vi "Scope_5782_Dual_PID_2channel.vi"() -> ()   [LabVIEW 2013]
uses:
  <vilib>/userdefined/High Color/nirio_resource_hc.ctl
  FPGA/DataMode.ctl
  <vilib>/Analysis/4window.llb/windowTd.ctl
  Host/Scope/controls/power_spectrum_unit.ctl
  Host/Scope5782/Scope/controls/5782_trigger_type.ctl
  Host/Scope/controls/Data_calc_mode.ctl
  Host/Scope/controls/Data_display_mode.ctl
  Host/Scope/controls/Graph_references.ctl
  Host/Scope/controls/graph_controls.ctl
  Host/Scope/controls/Channel_select.ctl
  Host/Communication/response.ctl
  Host/Communication/driver_status.ctl
  Host/Communication/Driver/RemoteConnection/RemoteReferences.ctl
  Host/Communication/Driver/TcpServerDriver/TcpServerDriver.lvclass
  Host/Scope5782/Scope/controls/c_t_type.ctl
  Host/Scope/controls/ScopeMode.ctl
  FPGA/fpga_settings.ctl
  Host/Communication/global_stop.vi
  <vilib>/FPGAPlugInAG/PXIe-7975R/niLvFpga_Open_PXIe-7975R.vi
  <vilib>/rvi/interface/common/dynamic/niFpgaDynamicAddResources.vi
  <vilib>/rvi/interface/common/niFpgaWaitOnOcc.vi
  <vilib>/Utility/error.llb/Error Cluster From Error Code.vi
  <vilib>/rvi/errors/niLvFpgaAdjustHostInterfaceError.vi
  <vilib>/FPGAPlugInAG/Dynamic/niLvFpga_Close_Dynamic.vi
  <vilib>/rvi/interface/nirviOpenFPGA/nirviOpenFPGA.xnode
  FPGA Bitfiles/Dual_PID_2_channel_oCwf2AgGrXE.lvbitx
  <vilib>/rvi/interface/nirviReadWriteControl/nirviReadWriteControl.xnode
  Host/Scope5782/Config/FPGAref_5782.ctl
  <vilib>/rvi/FXPMathLib/FxpInterpret/XNode/nifxpmath_Interpret.xnode
  <vilib>/rvi/interface/nirviMethod/nirviMethod.xnode
  <vilib>/rvi/interface/nirviCloseFPGA/nirviCloseFPGA.xnode
  Host/Utilities/Ticker/Ticker.lvclass
  NiFpgaLv.dll
  <vilib>/rvi/interface/Simulation/niFpgaSimulationCallBeginRW.vi
  Host/Communication/Driver/RemoteConnection/RemoteConnection.lvclass
  <vilib>/FPGAPlugInAG/Dynamic/niLvFpga_WriteFifo_Dynamic.vi
  <vilib>/rvi/errors/niLvFpgaMergeErrorWithErrorCode.vi
  <vilib>/Analysis/NI_AALPro.lvlib
panel:
  in  "Output enabled":bool=TRUE
  in  "unwrap phase":bool
  in  "Kp AM":fxp<+/-,32,4> caption="Kp"
  in  "Kd/T AM":fxp<+/-,32,4> caption="Kd/T"
  in  "Ki*T AM":fxp<+/-,32,4> caption="Ki*T"
  in  "Feedback AM":bool caption="Feedback"
  in  "c(t) AM":bool
  in  "c(t) phase":bool
  in  "Kp":fxp<+/-,32,4>
  in  "Kd/T":fxp<+/-,32,4>
  in  "Ki*T":fxp<+/-,32,4>
  in  "Feedback":bool
  in  "b":fxp<+/-,16,2>
  in  "a":fxp<+/-,16,2>
  in  "Fequency [kHz]":dbl format="%#_8g"
  in  "#bins":i32=1 min=1 max=16
  in  "ch1 DC offset":dbl caption="DC offset\nChannel 1"
  in  "ch0 DC offset":dbl caption="DC offset\nChannel 0"
  in  "Output delay delta":dbl(slide) scale=0.0..6.0
  in  "Output delay":dbl(slide) scale=0.0..6.0
  in  "Chart length":i32=200000
  in  "Trigmode":enum32{"Triggered", "Continuous"}(radio)
  in  "Refence for phase":T1
  in  "Graph_refs":T2
  out "Lower chart":dbl[][](graph)
  out "Upper chart":dbl[][](graph)
  out "Lower graph":i16[][](graph)
  in  "Buffer":T4
  in  "Display":T5
  in  "Output mixer fequency [MHz]":dbl
  in  "Trigger":T6
  in  "Ch1 Q":bool
  in  "Ch1 I":bool
  in  "Ch0 Q":bool
  in  "Ch0 I":bool
  in  "Ch1":bool
  in  "Ch0":bool
  out "stop 2":bool
  in  "Zoom freq X":bool
  in  "Zoom freq Y":bool
  in  "Zoom time Y":bool
  in  "Zoom time X":bool
  in  "Unit":T7
  in  "Window":T8=1 items=["Rectangle"=0, "Hanning"=1, "Hamming"=2, "Blackman-Harris"=3, "Exact Blackman"=4, "Blackman"=5, "Flat Top"=6, "4 Term B-Harris "=7, "7 Term B-Harris"=8, "Low Sidelobe"=9, "Blackman Nuttall"=11, "Triangle"=30, "Bartlett-Hanning"=31, "Bohman"=32, "Parzen"=33, "Welch"=34, "Kaiser"=60, "Dolph-Chebyshev"=61, "Gaussian"=62]
  in  "Samples per 5782 record":i32
  in  "Phase offset (deg)":dbl
  in  "Fequency [MHz]":dbl format="%#_8g"
  in  "Mode":T9
  in  "Mixer freq [MHz]":dbl
  out "freqdata":cluster{"f0":dbl, "df":dbl, "magnitude":dbl[]}[](graph)
  out "Upper graph":i16[][](graph)
  in  "Rumode":bool
  in  "Singleshot":bool
  out "error IO":errorcluster
  in  "stop":bool
  in  "resource name":T10="RIO0"
  out "Clocking Option Configured?":bool
  out "Configured?":bool
  # "FPGA setup"
  # "V"
  # "V"
  # "Output delay"
  # "ns"
  # "Auto Zoom"
  # "Output delay delta"
  # "ps"
  # "Amplitude modulation"
  # "5782"
  # "Phase"
  # "Amplitude"
  # "Simulated data"
  # "FFT"
  # "Auto Zoom"
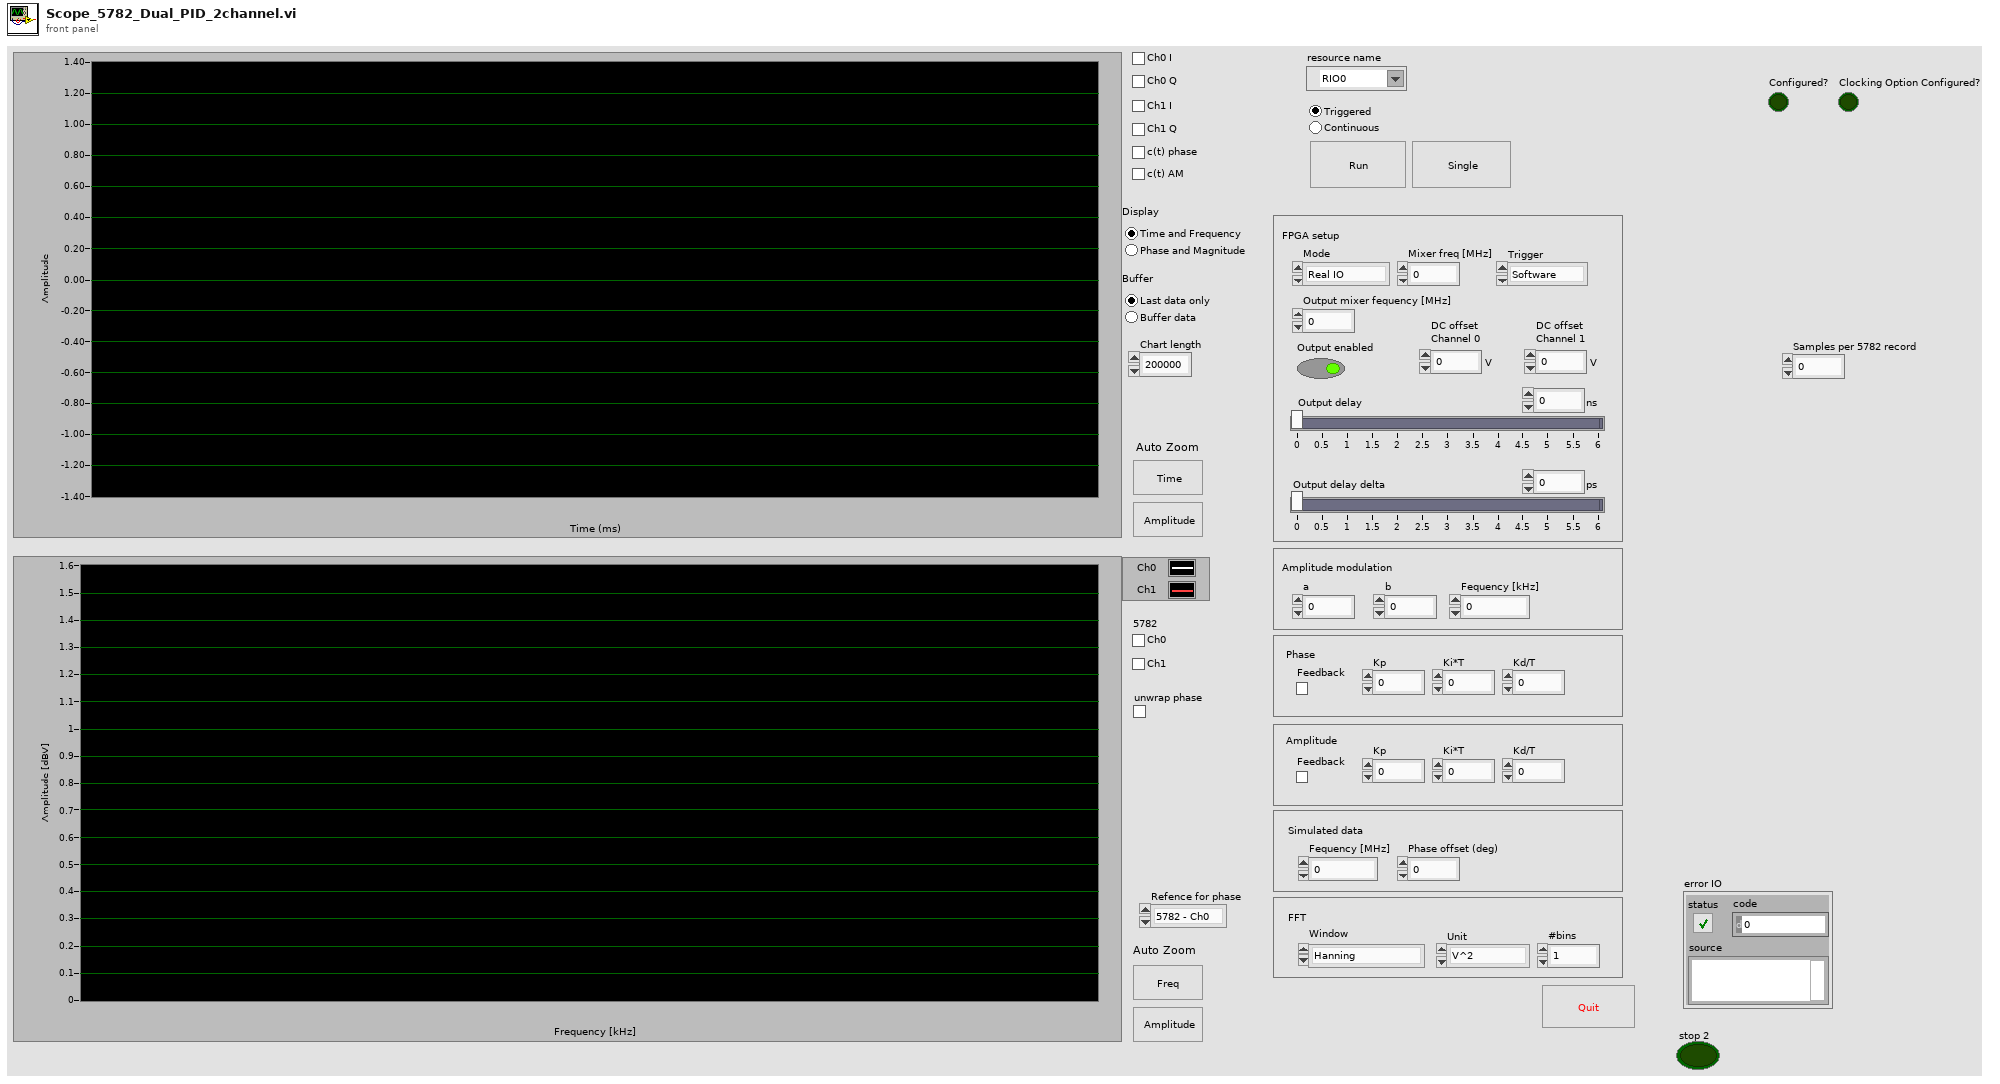
[diagram p1: front panel]
types:
  T1 = typedef "Channel_select.ctl" = enum16{"5782 - Ch0", "5782 - Ch1"}
  T2 = typedef "Graph_references.ctl" = cluster{"upper":T3, "lower":T3, "Freq graph":refnum<vi>}
  T3 = typedef "graph_controls.ctl" = cluster{"Graph":refnum<vi>, "Time btn":refnum<vi>, "Amplitude btn":refnum<vi>, "Chart":refnum<vi>}
  T4 = typedef "Data_display_mode.ctl" = enum32{"Last data only", "Buffer data"}
  T5 = typedef "Data_calc_mode.ctl" = enum32{"Time and Frequency", "Phase and Magnitude"}
  T6 = typedef "5782_trigger_type.ctl" = enum16{"Software", "Trigger input"}
  T7 = typedef "power_spectrum_unit.ctl" = enum16{"V^2", "V", "dBV"}
  T8 = typedef "NI_AALPro.lvlib/windowTd.ctl" = u32
  T9 = typedef "DataMode.ctl" = enum16{"Real IO", "Simulated"}
  T10 = typedef "nirio_resource_hc.ctl" = tag
  T11 = typedef "RemoteConnection.lvclass/RemoteReferences.ctl" = cluster{"a":refnum<vi>, "b":refnum<vi>, "fm":refnum<vi>, "Output delay":refnum<vi>, "Output delay delta":refnum<vi>}
  T12 = typedef "response.ctl" = cluster{"driver status":T13, "Sender":string, "Type":i32, "Variant":variant}
  T13 = typedef "driver_status.ctl" = enum16{"Normal", "Startup", "Connection lost", "Reconnected", "Timeout", "Idle", "Busy"}
  T14 = enum8{"Internal Clock PLL Off", "Internal Clock PLL On (REF IN)", "External Clock (CLK_IN)", "Internal Clock PLL On (IoModSyncClk)"}
  T15 = typedef "message_queue.ctl" = refnum<queue>
  T16 = typedef "FPGAref_5782.ctl" = refnum<k20>
  T17 = typedef "scope_params_5782.ctl" = cluster{"scope mode":T18, "ticker":refnum<class "Ticker.lvclass">, "samples per record":i32, "FPGA ref":T16, "data mode":T9, "5782 Trigger":T6, "Chart length":i32, "RemoteConnection":refnum<class "RemoteConnection.lvclass">, "last phase":dbl[]}
  T18 = typedef "ScopeMode.ctl" = enum16{"Stopped", "Single", "Running", "Continuous"}
  T19 = typedef "c_t_type.ctl" = enum16{"Phase", "AM", "Both", "None"}
  T20 = typedef "fpga_settings.ctl" = enum16{"Feedback Enable", "New FIR coeffs", "FIR shift", "Enable filter", "Set Downsample", "Downsample", "CIC Gain", "Record length", "Trigger samples", "Quiet time", "a_am", "b_am", "Use fixed delay", "fixed sin_fi", "fixed cos_fi", "Ki*Tau", "Kp", "Kd_Tau", "Fi_start", "Fi_delta", "DC_offs 0", "DC_offs 1", "Ki*Tau am", "Kp am", "Kd_Tau am", "Feedback AM"}
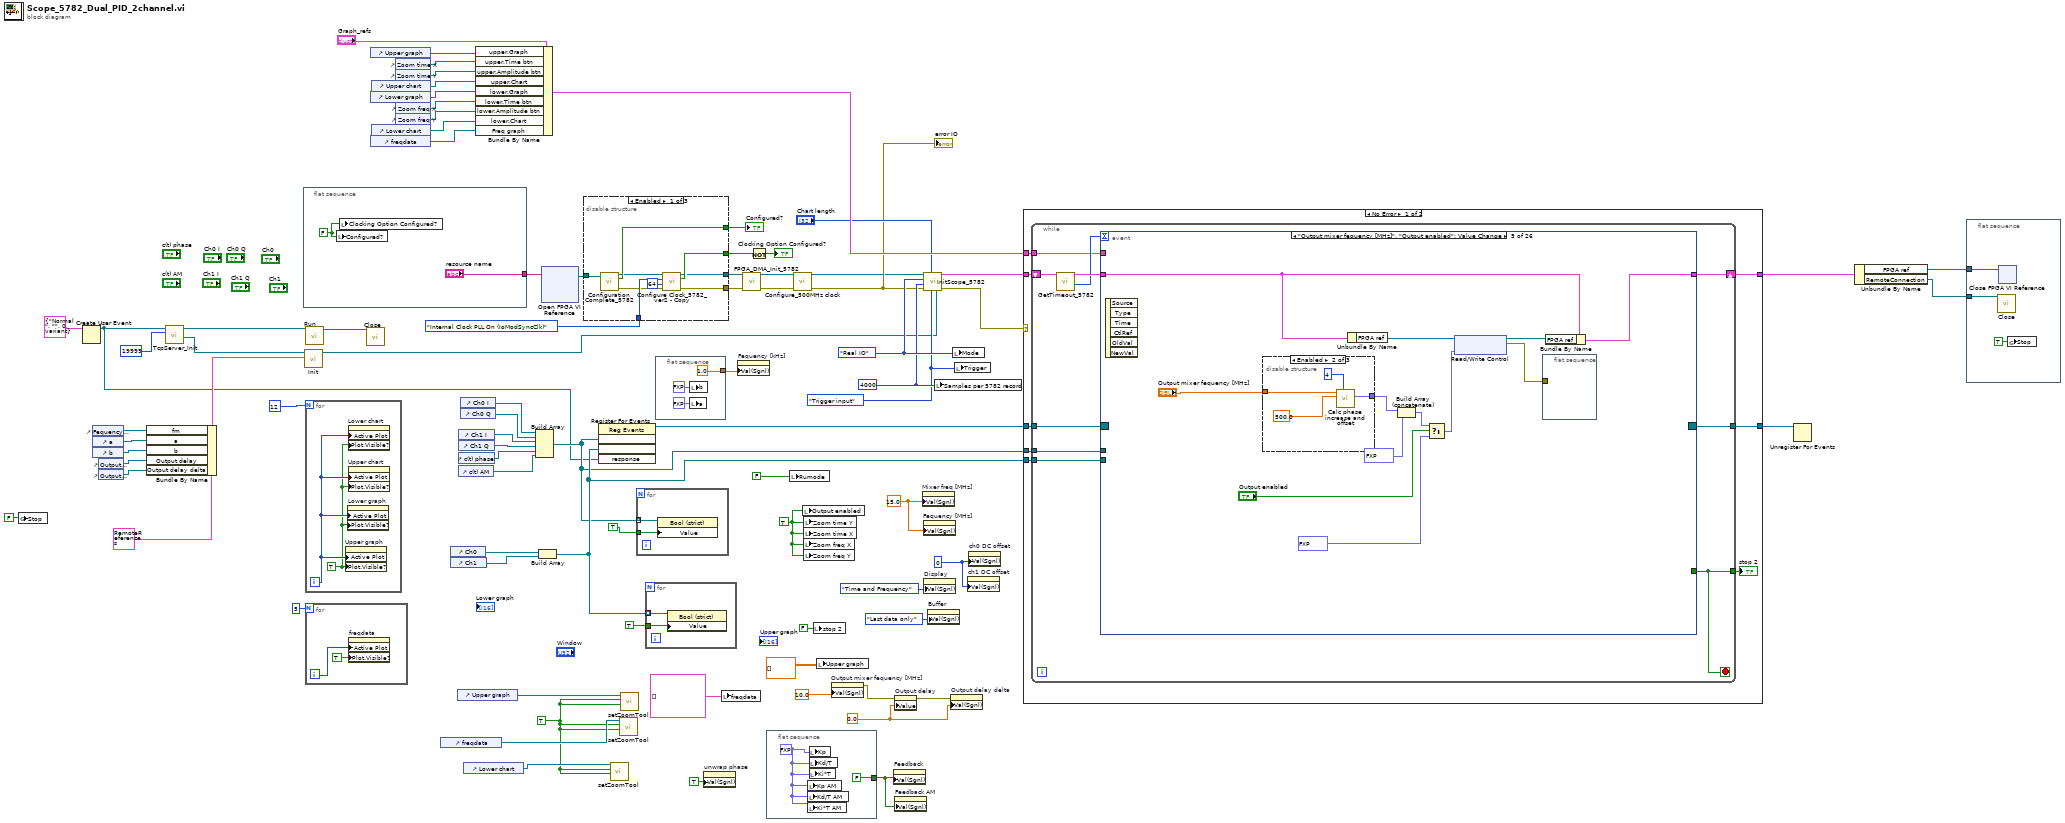
[diagram p0: block diagram]
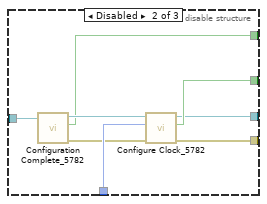
[diagram p2: hidden frame]
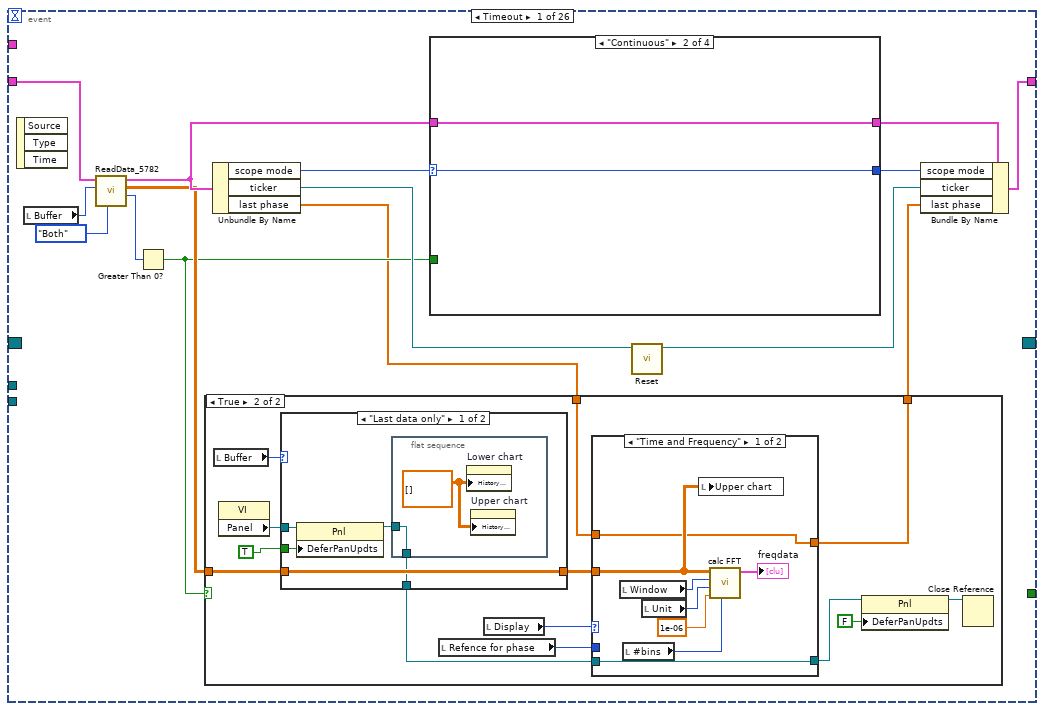
[diagram p4: hidden frame]
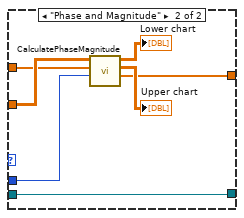
[diagram p7: hidden frame]
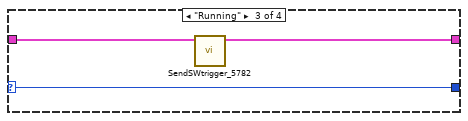
[diagram p9: hidden frame]
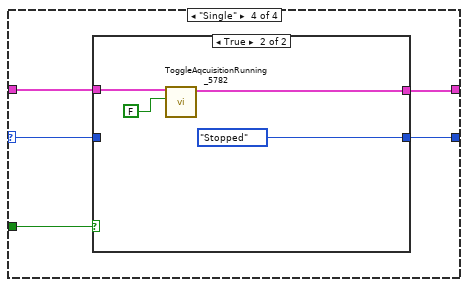
[diagram p10: hidden frame]
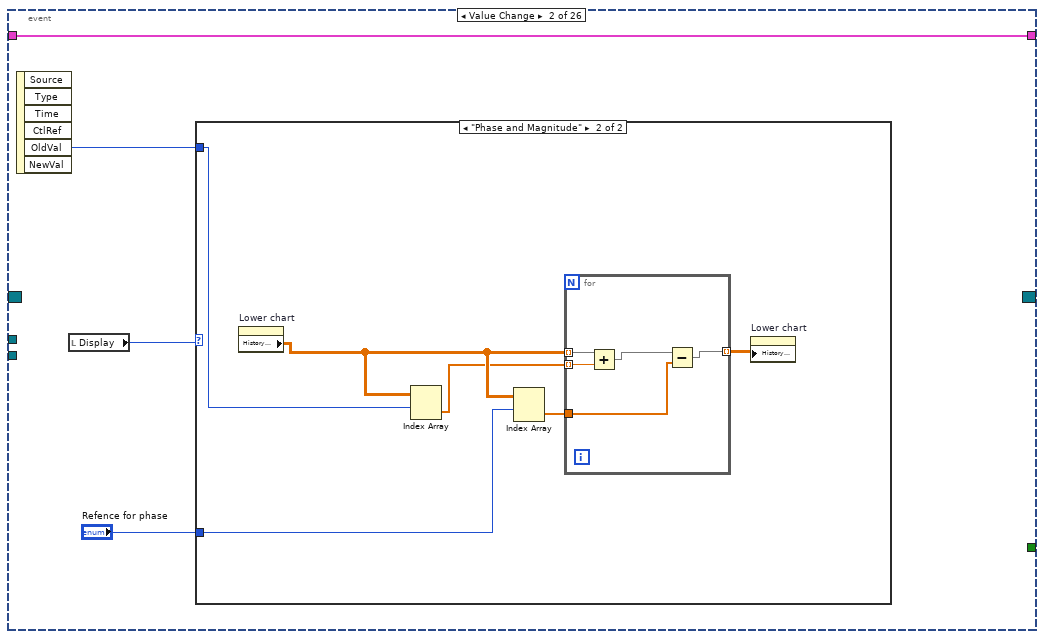
[diagram p12: hidden frame]
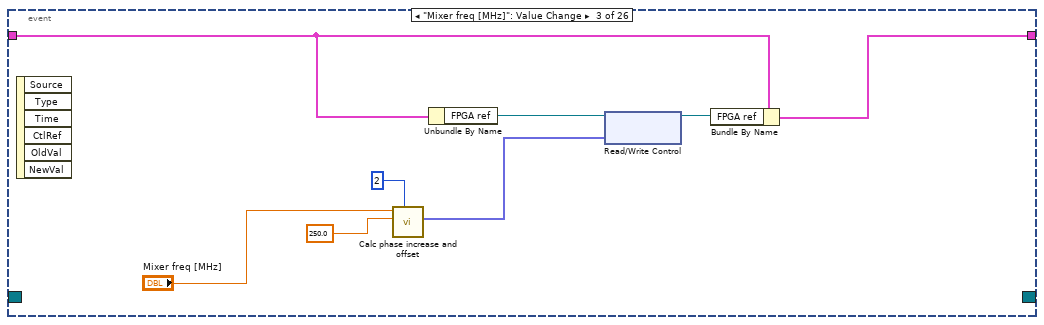
[diagram p14: hidden frame]
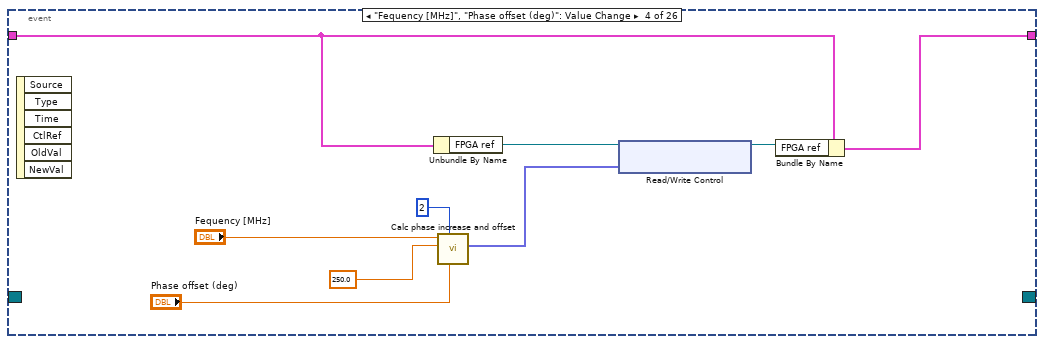
[diagram p15: hidden frame]
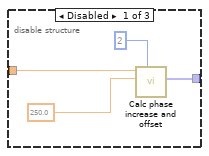
[diagram p16: hidden frame]
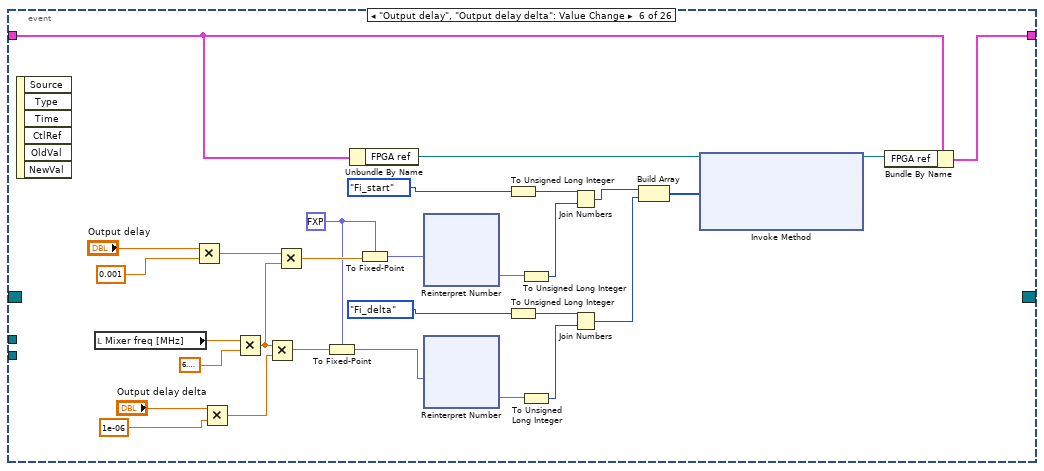
[diagram p18: hidden frame]
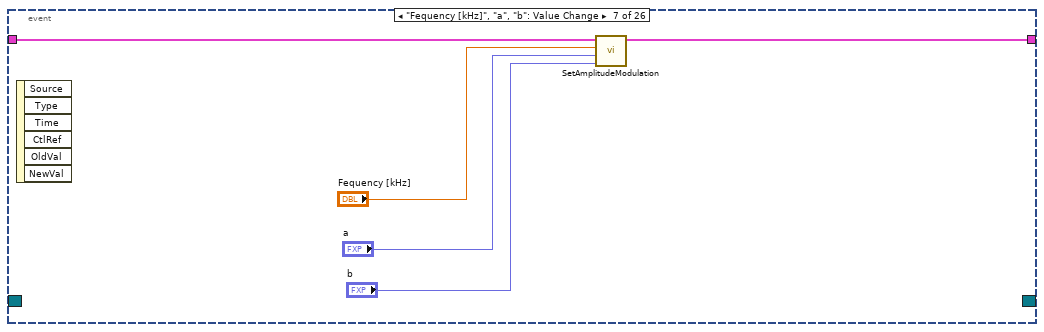
[diagram p19: hidden frame]
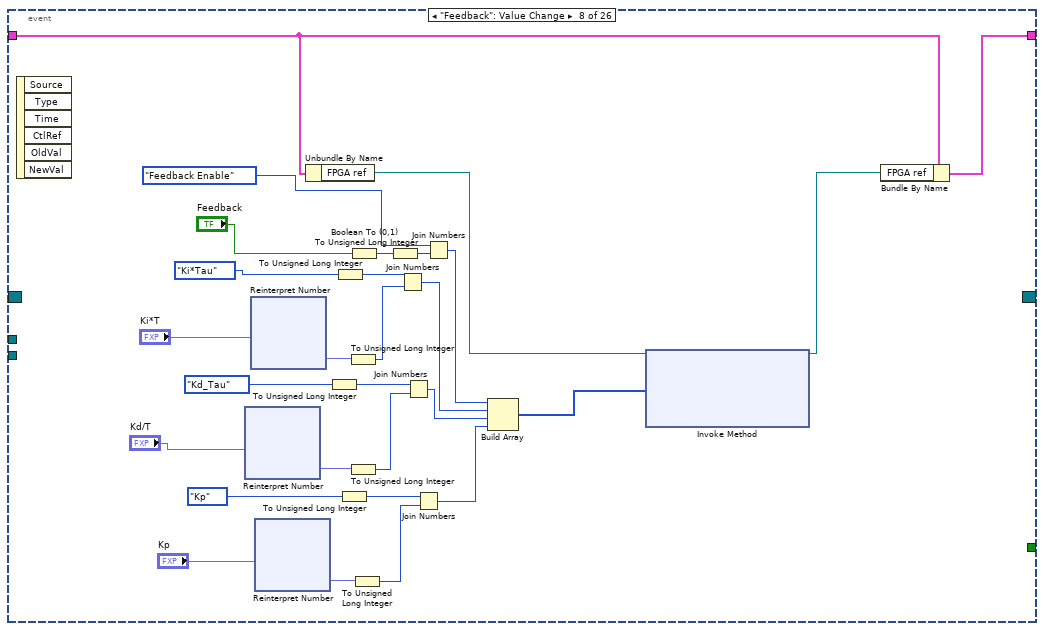
[diagram p20: hidden frame]
diagram:
  w31 = i16 0 ("Value (Signaling)")
  w32 = 0.0 ("Value (Signaling)")
  w55 = 5782_trigger_type."Trigger input" ("Trigger")
  w13 = TRUE ("Zoom  X")
  w1 = TRUE ("Rumode")
  w68 = DataMode."Real IO" ("Mode")
  w57 = 4000 ("Samples to aqcuire")
  w79 = 15.0 ("Mixer requency [MHz]")
  n1 = global write "global_stop.vi" "Stop"(FALSE ("Stop")) -> ()
  n2 = Create User Event(user event datatype=T12 {"driver status"=enum."Normal", "Sender"="", "Type"=0, "Variant"=variant} ("response")) -> (user event=w19:refnum<user-event>)  [unwired: 1 in, 1 out]
  n3 = control-ref of="Fequency [kHz]"() -> (w21:refnum<vi>)
  n4 = control-ref of="a"() -> (w22:refnum<vi>)
  n5 = control-ref of="b"() -> (w20:refnum<vi>)
  n6 = control-ref of="Output delay"() -> (w4:refnum<vi>)
  n7 = control-ref of="Output delay delta"() -> (w3:refnum<vi>)
  n8 = Bundle By Name(cluster=T11 {"a"=refnum, "b"=refnum, "fm"=refnum, "Output delay"=refnum, "Output delay delta"=refnum} ("refs"), "fm"=w21, "a"=w22, "b"=w20, "Output delay"=w4, "Output delay delta"=w3) -> (w29:T11)
  n9 = call "TcpServer_Init.vi"("local port"=u16 19999, "response event"=w19) -> ("Message queue"=w27:T15, "TcpServerDriver"=w24:refnum<class "TcpServerDriver.lvclass">)  [unwired: 8 in]
  n10 = flat-sequence {
    tunnel: ["resource name"] -> w69
    frame #0 {
      w84 = FALSE ("Trigger Acquisition")
      n11 = local write "Configured?"(w84) -> ()
      n12 = local write "Clocking Option Configured?"(w84) -> ()
    }
  }
  n13 = call "Init.vi"("refs"=w29, "server queue"=w27) -> ("RemoteConnection"=w18:refnum<class "RemoteConnection.lvclass">)  [unwired: 9 in]
  n14 = for {
    N: 12 -> [_]
    i -> [w87]
    w86 = TRUE ("Plot.Visible")
    n15 = property on="Upper graph" class="WFGraph (strict)"("Active Plot"=w87, "Plot.Visible?"=w86) -> ()  [unwired: 2 in, 2 out]
    n16 = property on="Lower graph" class="WFGraph (strict)"("Active Plot"=w87, "Plot.Visible?"=w86) -> ()  [unwired: 2 in, 2 out]
    n17 = property on="Lower chart" class="WFChart (strict)"("Active Plot"=w87, "Plot.Visible?"=w86) -> ()  [unwired: 2 in, 2 out]
    n18 = property on="Upper chart" class="WFChart (strict)"("Active Plot"=w87, "Plot.Visible?"=w86) -> ()  [unwired: 2 in, 2 out]
  }
  n19 = for {
    N: 5 -> [_]
    i -> [w88]
    n20 = property on="freqdata" class="WFGraph (strict)"("Active Plot"=w88, "Plot.Visible?"=TRUE ("Plot.Visible")) -> ()  [unwired: 2 in, 2 out]
  }
  n21 = call-dynamic "Run.vi"("BaseDriver in"=w24) -> ("BaseDriver out"=w25:refnum<class "TcpServerDriver.lvclass">)  [unwired: 9 in, 1 out]
  n22 = call-dynamic "Close.vi"("BaseDriver in"=w25) -> ()  [unwired: 9 in, 2 out]
  n23 = control-ref of="Upper graph"() -> (w52:refnum<vi>)
  n24 = control-ref of="Lower graph"() -> (w48:refnum<vi>)
  n25 = control-ref of="freqdata"() -> (w44:refnum<vi>)
  n26 = control-ref of="Upper chart"() -> (w49:refnum<vi>)
  n27 = control-ref of="Lower chart"() -> (w45:refnum<vi>)
  n28 = control-ref of="Zoom time X"() -> (w51:refnum<vi>)
  n29 = control-ref of="Zoom time Y"() -> (w50:refnum<vi>)
  n30 = control-ref of="Zoom freq X"() -> (w47:refnum<vi>)
  n31 = control-ref of="Zoom freq Y"() -> (w46:refnum<vi>)
  n32 = control-ref of="freqdata"() -> (w58:refnum<vi>)
  n33 = control-ref of="Ch0"() -> (w65:refnum<vi>)
  n34 = control-ref of="Ch1"() -> (w66:refnum<vi>)
  n35 = control-ref of="Upper graph"() -> (w59:refnum<vi>)
  n36 = control-ref of="c(t) AM"() -> (w6:refnum<vi>)
  n37 = control-ref of="Ch1 I"() -> (w63:refnum<vi>)
  n38 = control-ref of="Ch1 Q"() -> (w64:refnum<vi>)
  n39 = control-ref of="c(t) phase"() -> (w7:refnum<vi>)
  n40 = control-ref of="Ch0 I"() -> (w61:refnum<vi>)
  n41 = control-ref of="Ch0 Q"() -> (w62:refnum<vi>)
  n42 = control-ref of="Lower chart"() -> (w14:refnum<vi>)
  n43 = Bundle By Name(cluster="Graph_refs", "upper.Graph"=w52, "upper.Time btn"=w51, "upper.Amplitude btn"=w50, "upper.Chart"=w49, "lower.Graph"=w48, "lower.Time btn"=w47, "lower.Amplitude btn"=w46, "lower.Chart"=w45, "Freq graph"=w44) -> (w43:T2)
  n44 = Build Array(w61, w62, w63, w64, w7, w6) -> (w60:refnum<vi>[])
  n45 = Build Array(w65, w66) -> (w71:refnum<vi>[])
  n46 = xnode "Open FPGA VI Reference"("resource name"=w69) -> ("FPGA VI Reference Out"=w37:refnum<k20>)  [unwired: 1 in, 1 out]
  n47 = disable-structure shown="Enabled" {
    disable-tunnel: [w98 w106 _] -> w39
    disable-tunnel: T14."Internal Clock PLL On (IoModSyncClk)" ("Clock Source") -> [w97 w105 _]
    disable-tunnel: [w95 w103 _] -> w38
    disable-tunnel: [w94 w100 w107] -> w12
    disable-tunnel: w37 -> [w92 w102 w107]
    disable-tunnel: [w93 w99 _] -> w35
    frame Enabled {
      n48 = call "Configuration Complete_5782.vi"("FPGA VI Reference in"=w92) -> ("error out"=w96:errorcluster, "Configured?"=w93:bool, "FPGA VI Reference out"=w91:refnum<k20>)  [unwired: 8 in]
      n49 = call "Configure Clock_5782_ver2 - Copy.vi"("error in"=w96, "User Data 1"=u8 64, "Clock Source"=w97, "FPGA VI Reference"=w91) -> ("error out"=w95:errorcluster, "Configuration Error"=w98:bool, "FPGA VI Reference out"=w94:refnum<k20>)  [unwired: 5 in]
    }
    frame Disabled {
      n50 = call "Configuration Complete_5782.vi"("FPGA VI Reference in"=w102) -> ("error out"=w104:errorcluster, "Configured?"=w99:bool, "FPGA VI Reference out"=w101:refnum<k20>)  [unwired: 8 in]
      n51 = call "Configure Clock_5782.vi"("error in"=w104, "Clock Source"=w105, "FPGA VI Reference in"=w101) -> ("error out"=w103:errorcluster, "Configuration Error"=w106:bool, "FPGA VI Reference Out"=w100:T16)  [unwired: 6 in]
    }
    frame Disabled {
    }
  }
  "Configured?" <- w35
  n52 = register-events(w60, w71, w19) -> (reference out=w75:refnum<event-registration>)  [unwired: 2 in, 1 out]
  n53 = call "setZoomTool.vi"("Zoom Y"=w13, "Zoom  X"=w13, "reference"=w14) -> ()  [unwired: 9 in]
  n54 = call "setZoomTool.vi"("Zoom Y"=w13, "Zoom  X"=w13, "reference"=w58) -> ()  [unwired: 9 in]
  n55 = call "setZoomTool.vi"("Zoom Y"=w13, "Zoom  X"=w13, "reference"=w59) -> ()  [unwired: 9 in]
  n56 = for {
    tunnel: w60 -> [w109] mode=indexing
    tunnel: TRUE ("Rumode") -> [w108]
    n57 = property class="Bool (strict)"(reference=w109, "Value"=w108) -> ()  [unwired: 1 in, 2 out]
  }
  n58 = for {
    tunnel: w71 -> [w111] mode=indexing
    tunnel: TRUE ("Rumode") -> [w110]
    n59 = property class="Bool (strict)"(reference=w111, "Value"=w110) -> ()  [unwired: 1 in, 2 out]
  }
  n60 = flat-sequence {
    tunnel: [1.0 ("Value (Signaling)")] -> w30
    frame #0 {
      n61 = local write "b"(fxp<+/-,16,2> 0.0 ("b")) -> ()
      n62 = local write "a"(fxp<+/-,16,2> 1.0 ("a")) -> ()
    }
  }
  n63 = property on="unwrap phase" class="Bool (strict)"("Val(Sgnl)"=TRUE ("Value (Signaling)")) -> ()  [unwired: 2 in, 2 out]
  n64 = local write "freqdata"(cluster{"f0":dbl, "df":dbl, "magnitude":dbl[]}[] [] ("freqdata")) -> ()
  n65 = property on="Fequency [kHz]" class="DigNum (strict)"("Val(Sgnl)"=w30) -> ()  [unwired: 2 in, 2 out]
  n66 = call "FPGA_DMA_Init_5782.vi"("error in (no error)"=w38, "FPGA VI Reference"=w12) -> ("error out"=w10:errorcluster, "FPGA VI Out"=w11:refnum<k20>)  [unwired: 7 in, 1 out]
  n67 = Not(x=w39) -> (.not. x?=→"Clocking Option Configured?":bool)
  n68 = flat-sequence {
    tunnel: [FALSE] -> w5
    frame #0 {
      w115 = fxp<+/-,32,4> 0.0 ("Kp")
      n69 = local write "Kp AM"(w115) -> ()
      n70 = local write "Kd/T AM"(w115) -> ()
      n71 = local write "Ki*T AM"(w115) -> ()
      n72 = local write "Kp"(w115) -> ()
      n73 = local write "Kd/T"(w115) -> ()
      n74 = local write "Ki*T"(w115) -> ()
    }
  }
  n75 = local write "Rumode"(FALSE ("Rumode")) -> ()
  n76 = call "Configure_500MHz clock.vi"("error in"=w10, "FPGA SPI config ref"=w11) -> ("error out"=w9:errorcluster, "FPGA SPI config out"=w8:refnum<k20>)  [unwired: 8 in]
  "error IO" <- w9
  n77 = local write "Output enabled"(w1) -> ()
  n78 = local write "Zoom time Y"(w1) -> ()
  n79 = local write "Zoom time X"(w1) -> ()
  n80 = local write "Zoom freq X"(w1) -> ()
  n81 = local write "Zoom freq Y"(w1) -> ()
  n82 = local write "stop 2"(FALSE ("stop 2")) -> ()
  n83 = local write "Upper graph"(dbl[][] [] ("Timedata")) -> ()
  n84 = property on="Output mixer fequency [MHz]" class="DigNum (strict)"("Val(Sgnl)"=10.0 ("Mixer requency [MHz]")) -> (error out=w33:errorcluster)  [unwired: 2 in, 1 out]
  n85 = property on="Feedback" class="Bool (strict)"("Val(Sgnl)"=w5) -> ()  [unwired: 2 in, 2 out]
  n86 = property on="Output delay" class="Slide (strict)"(error in=w33, "Value"=w32) -> (error out=w34:errorcluster)  [unwired: 1 in, 1 out]
  n87 = property on="Feedback AM" class="Bool (strict)"("Val(Sgnl)"=w5) -> ()  [unwired: 2 in, 2 out]
  n88 = property on="Mixer freq [MHz]" class="DigNum (strict)"("Val(Sgnl)"=w79) -> ()  [unwired: 2 in, 2 out]
  n89 = property on="Fequency [MHz]" class="DigNum (strict)"("Val(Sgnl)"=w79) -> ()  [unwired: 2 in, 2 out]
  n90 = call "InitScope_5782.vi"("RemoteConnection"=w18, "Trigger"=w55, "Chart length"="Chart length", "error in"=w9, "Samples Per Trigger"=w57, "data mode"=w68, "FPGA ref"=w8) -> ("error out"=w15:errorcluster, "scope params"=w83:T17)  [unwired: 3 in]
  n91 = property on="Display" class="RadioBtnsControl (strict)"("Val(Sgnl)"=Data_calc_mode."Time and Frequency" ("Value (Signaling)")) -> ()  [unwired: 2 in, 2 out]
  n92 = property on="Buffer" class="RadioBtnsControl (strict)"("Val(Sgnl)"=enum32{"Last data only", "Buffer data"}."Last data only" ("Value (Signaling)")) -> ()  [unwired: 2 in, 2 out]
  n93 = local write "Samples per 5782 record"(w57) -> ()
  n94 = property on="Output delay delta" class="Slide (strict)"(error in=w34, "Val(Sgnl)"=w32) -> ()  [unwired: 1 in, 2 out]
  n95 = local write "Mode"(w68) -> ()
  n96 = local write "Trigger"(w55) -> ()
  n97 = property on="ch1 DC offset" class="DigNum (strict)"("Val(Sgnl)"=w31) -> ()  [unwired: 2 in, 2 out]
  n98 = property on="ch0 DC offset" class="DigNum (strict)"("Val(Sgnl)"=w31) -> ()  [unwired: 2 in, 2 out]
  n99 = case shown="No Error" w15 {
    tunnel: w83 -> [w124 w498]
    tunnel: [w123 w498] -> w56
    tunnel: w75 -> [w122 w497]
    tunnel: [w121 w497] -> w74
    tunnel: w60 -> [w120 _]
    tunnel: w71 -> [w119 _]
    tunnel: w43 -> [w117 _]
    frame No Error {
      n100 = while {
        shift-right: [w134] -> w123
        shift-left: w124 -> [w133]
        tunnel: w122 -> [w130]
        tunnel: [w129] -> w121
        tunnel: w120 -> [w128]
        tunnel: w119 -> [w127]
        tunnel: [w126] -> w118
        tunnel: w117 -> [w125]
        stop <- w126 stop-if-true
        n101 = call "GetTimeout_5782.vi"("scope in"=w133) -> ("Time left"=w131:i32, "scope out"=w132:T17)  [unwired: 9 in]
        n102 = event shown="[4] \"Output mixer fequency [MHz]\", \"Output enabled\": Value Change" {
          selector: w130 -> [_ _ _ _ _ _ _ _ _ _ _ _ _ _ _ _ _ _ _ _ _ _ _ _ _ _]
          dyn-events: [_ _ _ _ _ _ _ _ _ _ _ _ _ _ _ _ _ _ _ _ _ _ _ _ _ _] -> w129
          timeout: w131 -> [_ _ _ _ _ _ _ _ _ _ _ _ _ _ _ _ _ _ _ _ _ _ _ _ _ _]
          tunnel: [_ _ _ _ _ _ _ _ _ _ _ _ _ _ _ _ _ _ _ _ "stop" _ _ _ _ _] -> w126
          tunnel: w132 -> [w144 w209 w227 w233 w249 w284 w291 w319 w347 w361 w375 w379 w383 w386 w396 w404 w429 w440 w453 w458 w461 w468 w478 w483 w489 w496]
          tunnel: [w147 w209 w225 w232 w248 w283 w290 w318 w346 w360 w374 w378 w382 w385 w393 w401 w429 w440 w453 w457 w461 w468 w478 w483 w489 w496] -> w134
          tunnel: w128 -> [_ _ _ _ _ _ _ _ _ _ _ _ _ _ _ _ w428 _ _ _ _ _ _ _ _ _]
          tunnel: w127 -> [_ _ _ _ _ _ _ _ _ _ _ _ _ _ _ _ _ w430 _ _ _ _ _ _ _ _]
          tunnel: w125 -> [_ _ _ _ _ _ _ _ _ _ _ _ _ _ _ _ _ _ _ _ _ _ _ _ _ w493]
          event Timeout {
            n103 = event-data() -> ()  [unwired: 1 in, 3 out]
            n104 = local read "Buffer"() -> (w138:T4)
            n105 = call "ReadData_5782.vi"("c(t)"=c_t_type."Both", "Buffer mode"=w138, "scope params"=w144) -> ("Num elements"=w140:i32, "data"=w141:dbl[][], "scope params out"=w143:T17)  [unwired: 6 in]
            n106 = Greater Than 0?(x=w140) -> (x > 0?=w139:bool)
            n107 = Unbundle By Name(w143) -> ("scope mode"=w146:T18, "ticker"=w149:refnum<class "Ticker.lvclass">, "last phase"=w137:dbl[])
            n108 = case shown="True" w139 {
              tunnel: w141 -> [_ w160]
              tunnel: w137 -> [w150 w152]
              tunnel: [w150 w151] -> w136
              frame False {
              }
              frame True {
                n109 = local read "Buffer"() -> (w162:T4)
                n110 = property class="VI"() -> ("Panel"=w155:refnum<vi>)  [unwired: 2 in, 2 out]
                n111 = case shown="\"Last data only\"" w162 {
                  tunnel: w160 -> [w168 w172]
                  tunnel: [w168 w172] -> w161
                  tunnel: w155 -> [w167 w171]
                  tunnel: TRUE ("Defer Panel Updates") -> [w165 _]
                  tunnel: [w164 w171] -> w153
                  frame "Last data only" {
                    n112 = property class="Pnl"(reference=w167, "DeferPanUpdts"=w165) -> (reference out=w166:refnum<vi>)  [unwired: 1 in, 1 out]
                    n113 = flat-sequence {
                      tunnel: w166 -> [w169]
                      tunnel: [w169] -> w164
                      frame #0 {
                        w170 = dbl[][] [] ("History Data")
                        n114 = property on="Lower chart" class="WFChart (strict)"("History Data"=w170) -> ()  [unwired: 2 in, 2 out]
                        n115 = property on="Upper chart" class="WFChart (strict)"("History Data"=w170) -> ()  [unwired: 2 in, 2 out]
                      }
                    }
                  }
                  frame "Buffer data" {
                  }
                }
                n116 = local read "Refence for phase"() -> (w159:T1)
                n117 = local read "Display"() -> (w163:T5)
                n118 = case shown="\"Time and Frequency\"" w163 {
                  tunnel: w161 -> [w176 w187]
                  tunnel: w159 -> [_ w184]
                  tunnel: [w175 w183] -> w157
                  tunnel: w153 -> [w175 w183]
                  tunnel: w152 -> [w173 w182]
                  tunnel: [w173 w181] -> w151
                  frame "Time and Frequency" {
                    n119 = local read "Window"() -> (w177:T8)
                    n120 = local read "#bins"() -> (w174:i32)
                    n121 = local read "Unit"() -> (w178:T7)
                    n122 = local write "Upper chart"(w176) -> ()
                    n123 = call "calc FFT.vi"("#bins"=w174, "dt"=1e-06, "Unit"=w178, "Window"=w177, "data"=w176) -> ("Power Spectrum / PSD"=→"freqdata":cluster{"f0":dbl, "df":dbl, "magnitude":dbl[]}[])  [unwired: 6 in]
                  }
                  frame "Phase and Magnitude" {
                    n124 = call "CalculatePhaseMagnitude.vi"("phase reference channel"=w184, "previous phase"=w182, "data"=w187) -> ("last phase"=w181:dbl[], "Magnitude"=→"Upper chart":dbl[][], "Phase"=→"Lower chart":dbl[][])  [unwired: 6 in]
                  }
                }
                n125 = property class="Pnl"(reference=w157, "DeferPanUpdts"=FALSE ("Defer Panel Updates")) -> (reference out=w156:refnum<vi>)  [unwired: 1 in, 1 out]
                n126 = Close Reference(reference=w156) -> ()  [unwired: 1 in, 1 out]
              }
            }
            n127 = case shown="\"Continuous\"" w146 {
              selector: w146 -> [w189 w191 w194 w195]
              tunnel: [w189 w191 w194 w199] -> w145
              tunnel: w143 -> [w188 w190 w193 w197]
              tunnel: [w188 w190 w192 w196] -> w142
              tunnel: w139 -> [_ _ _ w198]
              frame "Stopped" {
              }
              frame "Continuous" {
              }
              frame "Running" {
                n128 = call "SendSWtrigger_5782.vi"("scope in"=w193) -> ("scope out"=w192:T17)  [unwired: 9 in, 1 out]
              }
              frame "Single" {
                n129 = case shown="True" w198 {
                  tunnel: [w200 ScopeMode."Stopped" ("scope mode")] -> w199
                  tunnel: w197 -> [w201 w204]
                  tunnel: [w201 w203] -> w196
                  tunnel: w195 -> [w200 _]
                  frame False {
                  }
                  frame True {
                    n130 = call "ToggleAqcuisitionRunning_5782.vi"("Acquisition running"=FALSE, "scope in"=w204) -> ("scope out"=w203:T17)  [unwired: 8 in, 1 out]
                  }
                }
              }
            }
            n131 = call "Reset.vi"("Ticker in"=w149) -> ("Ticker out"=w148:refnum<class "Ticker.lvclass">)  [unwired: 9 in, 1 out]
            n132 = Bundle By Name(cluster=w142, "scope mode"=w145, "ticker"=w148, "last phase"=w136) -> (w147:T17)
          }
          event Value Change {
            n133 = event-data() -> ("OldVal"=w206:T1)  [unwired: 1 in, 5 out]
            n134 = local read "Display"() -> (w207:T5)
            n135 = case shown="\"Phase and Magnitude\"" w207 {
              tunnel: "Refence for phase" -> [_ w214]
              tunnel: w206 -> [_ w212]
              frame "Time and Frequency", Default {
              }
              frame "Phase and Magnitude" {
                n136 = property on="Lower chart" class="WFChart (strict)"() -> ("History Data"=w213:dbl[][])  [unwired: 2 in, 2 out]
                n137 = Index Array(array=w213, index (row)=w212) -> (element=w211:dbl[])  [unwired: 1 in]
                n138 = Index Array(array=w213, index (row)=w214) -> (element=w215:dbl[])  [unwired: 1 in]
                n139 = for {
                  tunnel: w213 -> [w218] mode=indexing
                  tunnel: w215 -> [w220]
                  tunnel: [w219] -> w210 mode=indexing
                  tunnel: w211 -> [w217] mode=indexing
                  n140 = Add(x=w218, y=w217) -> (x+y=w216:dbl[])
                  n141 = Subtract(x=w216, y=w220) -> (x-y=w219:dbl[])
                }
                n142 = property on="Lower chart" class="WFChart (strict)"("History Data"=w210) -> ()  [unwired: 2 in, 2 out]
              }
            }
          }
          event "Mixer freq [MHz]": Value Change {
            n143 = event-data() -> ()  [unwired: 1 in, 6 out]
            n144 = call "Calc phase increase and offset.vi"("# of DDS"=2, "fclk (MHz)"=250.0 ("fclk (800MHz)"), "f_generated (MHz)"="Mixer freq [MHz]") -> ("Phase out"=w221:fxp<+,64,64>[])  [unwired: 6 in, 2 out]
            n145 = Unbundle By Name(w227) -> ("FPGA ref"=w228:T16)
            n146 = xnode "Read/Write Control"("FPGA VI Reference In"=w228, "Phase 5782"=w221) -> ("FPGA VI Reference Out"=w226:T16)  [unwired: 1 in, 1 out]
            n147 = Bundle By Name(cluster=w227, "FPGA ref"=w226) -> (w225:T17)
          }
          event "Fequency [MHz]", "Phase offset (deg)": Value Change {
            n148 = event-data() -> ()  [unwired: 1 in, 6 out]
            n149 = Unbundle By Name(w233) -> ("FPGA ref"=w235:T16)
            n150 = call "Calc phase increase and offset.vi"("Phase offset (deg)"="Phase offset (deg)", "# of DDS"=2, "fclk (MHz)"=250.0 ("fclk (800MHz)"), "f_generated (MHz)"="Fequency [MHz]") -> ("Phase out"=w229:fxp<+,64,64>[])  [unwired: 5 in, 2 out]
            n151 = xnode "Read/Write Control"("FPGA VI Reference In"=w235, "Simulated phase 5782"=w229) -> ("FPGA VI Reference Out"=w234:T16)  [unwired: 1 in, 1 out]
            n152 = Bundle By Name(cluster=w233, "FPGA ref"=w234) -> (w232:T17)
          }
          event "Output mixer fequency [MHz]", "Output enabled": Value Change {
            n153 = event-data() -> ()  [unwired: 1 in, 6 out]
            n154 = disable-structure shown="Enabled" {
              disable-tunnel: [w251 w255 _] -> w243
              disable-tunnel: "Output mixer fequency [MHz]" -> [w250 w254 _]
              frame Disabled {
                n155 = call "Calc phase increase and offset.vi"("# of DDS"=2, "fclk (MHz)"=250.0 ("fclk (800MHz)"), "f_generated (MHz)"=w250) -> ("Phase out"=w251:fxp<+,64,64>[])  [unwired: 6 in, 2 out]
              }
              frame Enabled {
                n156 = call "Calc phase increase and offset.vi"("# of DDS"=4, "fclk (MHz)"=500.0 ("fclk (800MHz)"), "f_generated (MHz)"=w254) -> ("Phase out"=w255:fxp<+,64,64>[])  [unwired: 6 in, 2 out]
              }
              frame Disabled {
              }
            }
            n157 = Unbundle By Name(w249) -> ("FPGA ref"=w245:T16)
            n158 = Build Array (concatenate)(w243, fxp<+,64,64>[] [0.0, 0.0, 0.0, 0.0] ("array")) -> (w239:fxp<+,64,64>[])
            n159 = Select(t=w239, s="Output enabled", f=fxp<+,64,64>[] [0.0, 0.0, 0.0, 0.0, 0.0, 0.0, 0.0, 0.0]) -> (s? t:f=w238:fxp<+,64,64>[])
            n160 = xnode "Read/Write Control"("FPGA VI Reference In"=w245, "Phase output"=w238) -> ("FPGA VI Reference Out"=w244:T16, "error out"=w246:errorcluster)  [unwired: 1 in]
            n161 = flat-sequence {
              tunnel: w246 -> [_]
              frame #0 {
              }
            }
            n162 = Bundle By Name(cluster=w249, "FPGA ref"=w244) -> (w248:T17)
          }
          event "Output delay", "Output delay delta": Value Change {
            w263 = fxp<+/-,32,4> 0.0 ("x")
            n163 = event-data() -> ()  [unwired: 1 in, 6 out]
            n164 = local read "Mixer freq [MHz]"() -> (w278:dbl)
            n165 = Multiply(x="Output delay", y=0.001) -> (x*y=w279:dbl)
            n166 = Multiply(x="Output delay delta", y=1e-06) -> (x*y=w281:dbl)
            n167 = Multiply(x=w278, y=6.283185307179586) -> (x*y=w276:dbl)
            n168 = Multiply(x=w276, y=w281) -> (x*y=w264:dbl)
            n169 = Multiply(x=w279, y=w276) -> (x*y=w266:dbl)
            n170 = To Fixed-Point(fixed-point type=w263, number=w264) -> (fixed-point=w262:fxp<+/-,32,4>)
            n171 = Unbundle By Name(w284) -> ("FPGA ref"=w259:T16)
            n172 = To Fixed-Point(fixed-point type=w263, number=w266) -> (fixed-point=w265:fxp<+/-,32,4>)
            n173 = xnode "Reinterpret Number"("x"=w265) -> ("y"=w272:fxp<+,32,32>)
            n174 = xnode "Reinterpret Number"("x"=w262) -> ("y"=w271:fxp<+,32,32>)
            n175 = To Unsigned Long Integer(number=fpga_settings."Fi_start" ("FPGA Setting")) -> (unsigned 32bit integer=w275:u32)
            n176 = To Unsigned Long Integer(number=fpga_settings."Fi_delta" ("FPGA Setting")) -> (unsigned 32bit integer=w268:u32)
            n177 = To Unsigned Long Integer(number=w272) -> (unsigned 32bit integer=w274:u32)
            n178 = To Unsigned Long Integer(number=w271) -> (unsigned 32bit integer=w269:u32)
            n179 = Join Numbers(hi=w275, lo=w274) -> ((hi.lo)=w260:u64)
            n180 = Join Numbers(hi=w268, lo=w269) -> ((hi.lo)=w261:u64)
            n181 = Build Array(w260, w261) -> (w267:u64[])
            n182 = xnode "Invoke Method"("FPGA VI Reference In"=w259, "Data"=w267) -> ("FPGA VI Reference Out"=w258:T16)  [unwired: 2 in, 2 out]
            n183 = Bundle By Name(cluster=w284, "FPGA ref"=w258) -> (w283:T17)
          }
          event "Fequency [kHz]", "a", "b": Value Change {
            n184 = event-data() -> ()  [unwired: 1 in, 6 out]
            n185 = call "SetAmplitudeModulation.vi"("b_am"="b", "a_am"="a", "Am freq [kHz]"="Fequency [kHz]", "scope in"=w291) -> ("scope out"=w290:T17)  [unwired: 7 in]
          }
          event "Feedback": Value Change {
            n186 = event-data() -> ()  [unwired: 1 in, 6 out]
            n187 = xnode "Reinterpret Number"("x"="Kd/T") -> ("y"=w305:fxp<+,32,32>)
            n188 = xnode "Reinterpret Number"("x"="Ki*T") -> ("y"=w302:fxp<+,32,32>)
            n189 = xnode "Reinterpret Number"("x"="Kp") -> ("y"=w309:fxp<+,32,32>)
            n190 = Unbundle By Name(w319) -> ("FPGA ref"=w317:T16)
            n191 = To Unsigned Long Integer(number=fpga_settings."Kd_Tau" ("FPGA Setting")) -> (unsigned 32bit integer=w303:u32)
            n192 = To Unsigned Long Integer(number=fpga_settings."Ki*Tau" ("FPGA Setting")) -> (unsigned 32bit integer=w299:u32)
            n193 = To Unsigned Long Integer(number=fpga_settings."Kp" ("FPGA Setting")) -> (unsigned 32bit integer=w306:u32)
            n194 = To Unsigned Long Integer(number=w302) -> (unsigned 32bit integer=w298:u32)
            n195 = To Unsigned Long Integer(number=w305) -> (unsigned 32bit integer=w304:u32)
            n196 = Boolean To (0,1)(Boolean="Feedback") -> (0, 1=w314:i16)
            n197 = To Unsigned Long Integer(number=w309) -> (unsigned 32bit integer=w308:u32)
            n198 = To Unsigned Long Integer(number=w314) -> (unsigned 32bit integer=w311:u32)
            n199 = Join Numbers(hi=w299, lo=w298) -> ((hi.lo)=w297:u64)
            n200 = Join Numbers(hi=w303, lo=w304) -> ((hi.lo)=w296:u64)
            n201 = Join Numbers(hi=w306, lo=w308) -> ((hi.lo)=w316:u64)
            n202 = Join Numbers(hi=fpga_settings."Feedback Enable" ("FPGA Setting"), lo=w311) -> ((hi.lo)=w312:u64)
            n203 = Build Array(w312, w297, w296, w316) -> (w315:u64[])
            n204 = xnode "Invoke Method"("FPGA VI Reference In"=w317, "Data"=w315) -> ("FPGA VI Reference Out"=w292:T16)  [unwired: 2 in, 2 out]
            n205 = Bundle By Name(cluster=w319, "FPGA ref"=w292) -> (w318:T17)
          }
          event "Feedback AM": Value Change {
            n206 = event-data() -> ()  [unwired: 1 in, 6 out]
            n207 = xnode "Reinterpret Number"("x"="Kd/T AM") -> ("y"=w334:fxp<+,32,32>)
            n208 = xnode "Reinterpret Number"("x"="Ki*T AM") -> ("y"=w331:fxp<+,32,32>)
            n209 = xnode "Reinterpret Number"("x"="Kp AM") -> ("y"=w338:fxp<+,32,32>)
            n210 = Unbundle By Name(w347) -> ("FPGA ref"=w345:T16)
            n211 = To Unsigned Long Integer(number=fpga_settings."Kd_Tau am" ("FPGA Setting")) -> (unsigned 32bit integer=w332:u32)
            n212 = To Unsigned Long Integer(number=fpga_settings."Ki*Tau am" ("FPGA Setting")) -> (unsigned 32bit integer=w330:u32)
            n213 = To Unsigned Long Integer(number=fpga_settings."Kp am" ("FPGA Setting")) -> (unsigned 32bit integer=w335:u32)
            n214 = To Unsigned Long Integer(number=w331) -> (unsigned 32bit integer=w329:u32)
            n215 = To Unsigned Long Integer(number=w334) -> (unsigned 32bit integer=w333:u32)
            n216 = Boolean To (0,1)(Boolean="Feedback AM") -> (0, 1=w342:i16)
            n217 = To Unsigned Long Integer(number=w338) -> (unsigned 32bit integer=w337:u32)
            n218 = To Unsigned Long Integer(number=w342) -> (unsigned 32bit integer=w339:u32)
            n219 = Join Numbers(hi=w330, lo=w329) -> ((hi.lo)=w328:u64)
            n220 = Join Numbers(hi=w332, lo=w333) -> ((hi.lo)=w327:u64)
            n221 = Join Numbers(hi=w335, lo=w337) -> ((hi.lo)=w344:u64)
            n222 = Join Numbers(hi=fpga_settings."Feedback AM" ("FPGA Setting"), lo=w339) -> ((hi.lo)=w340:u64)
            n223 = Build Array(w340, w328, w327, w344) -> (w343:u64[])
            n224 = xnode "Invoke Method"("FPGA VI Reference In"=w345, "Data"=w343) -> ("FPGA VI Reference Out"=w324:T16)  [unwired: 2 in, 2 out]
            n225 = Bundle By Name(cluster=w347, "FPGA ref"=w324) -> (w346:T17)
          }
          event "ch0 DC offset": Value Change {
            n226 = event-data() -> ()  [unwired: 1 in, 6 out]
            n227 = Unbundle By Name(w361) -> ("FPGA ref"=w349:T16)
            n228 = Divide(x=32768, y=5) -> (x/y=w358:dbl)
            n229 = Multiply(x="ch0 DC offset", y=w358) -> (x*y=w357:dbl)
            n230 = Round To Nearest(number=w357) -> (nearest integer value=w356:dbl)
            n231 = To Word Integer(number=w356) -> (16bit integer=w350:i16)
            n232 = xnode "Reinterpret Number"("x"=w350) -> ("y"=w353:fxp<+/-,16,14>)
            n233 = xnode "Reinterpret Number"("x"=w353) -> ("y"=w352:fxp<+,16,16>)
            n234 = call "Write 16bit value.vi"("value"=w352, "FPGA Setting"=fpga_settings."DC_offs 0", "FPGA ref"=w349) -> ("FPGA ref out"=w348:T16)  [unwired: 7 in, 1 out]
            n235 = Bundle By Name(cluster=w361, "FPGA ref"=w348) -> (w360:T17)
          }
          event "ch1 DC offset": Value Change {
            n236 = event-data() -> ()  [unwired: 1 in, 6 out]
            n237 = Unbundle By Name(w375) -> ("FPGA ref"=w363:T16)
            n238 = Divide(x=32768, y=5) -> (x/y=w372:dbl)
            n239 = Multiply(x="ch1 DC offset", y=w372) -> (x*y=w371:dbl)
            n240 = Round To Nearest(number=w371) -> (nearest integer value=w370:dbl)
            n241 = To Word Integer(number=w370) -> (16bit integer=w364:i16)
            n242 = xnode "Reinterpret Number"("x"=w364) -> ("y"=w367:fxp<+/-,16,14>)
            n243 = xnode "Reinterpret Number"("x"=w367) -> ("y"=w366:fxp<+,16,16>)
            n244 = call "Write 16bit value.vi"("value"=w366, "FPGA Setting"=fpga_settings."DC_offs 1", "FPGA ref"=w363) -> ("FPGA ref out"=w362:T16)  [unwired: 7 in, 1 out]
            n245 = Bundle By Name(cluster=w375, "FPGA ref"=w362) -> (w374:T17)
          }
          event Value Change {
            n246 = event-data() -> ()  [unwired: 1 in, 6 out]
            n247 = Unbundle By Name(w379) -> ("FPGA ref"=w381:T16)
            n248 = property on="Rumode" class="Bool (strict)"("Val(Sgnl)"=FALSE ("Value (Signaling)")) -> ()  [unwired: 2 in, 2 out]
            n249 = xnode "Read/Write Control"("FPGA VI Reference In"=w381, "Mode"="Mode") -> ("FPGA VI Reference Out"=w380:T16)  [unwired: 1 in, 1 out]
            n250 = Bundle By Name(cluster=w379, "FPGA ref"=w380, "data mode"="Mode") -> (w378:T17)
          }
          event Value Change {
            n251 = event-data() -> ()  [unwired: 1 in, 6 out]
            n252 = Bundle By Name(cluster=w383, "5782 Trigger"="Trigger") -> (w382:T17)
          }
          event "Samples per 5782 record": Value Change {
            n253 = event-data() -> ()  [unwired: 1 in, 6 out]
            n254 = Unbundle By Name(w386) -> ("FPGA ref"=w389:T16)
            n255 = xnode "Read/Write Control"("FPGA VI Reference In"=w389, "5782 record length"="Samples per 5782 record") -> ("FPGA VI Reference Out"=w388:T16)  [unwired: 1 in, 1 out]
            n256 = Bundle By Name(cluster=w386, "FPGA ref"=w388, "samples per record"="Samples per 5782 record") -> (w385:T17)
          }
          event "Singleshot": Value Change {
            n257 = event-data() -> ()  [unwired: 1 in, 6 out]
            n258 = local write "Rumode"(FALSE ("Rumode")) -> ()
            n259 = Bundle By Name(cluster=w396, "scope mode"=ScopeMode."Single") -> (w391:T17)
            n260 = call "ToggleContinousMode.vi"("Cont Acquisition"=FALSE, "scope in"=w391) -> ("scope out"=w390:T17)  [unwired: 8 in, 1 out]
            n261 = call "ToggleAqcuisitionRunning_5782.vi"("Acquisition running"=TRUE, "scope in"=w390) -> ("scope out"=w394:T17)  [unwired: 8 in, 1 out]
            n262 = call "SendSWtrigger_5782.vi"("scope in"=w394) -> ("scope out"=w393:T17)  [unwired: 9 in, 1 out]
          }
          event "Rumode": Value Change {
            n263 = event-data() -> ()  [unwired: 1 in, 6 out]
            n264 = case shown="\"Triggered\"" "Trigmode" {
              tunnel: [ScopeMode."Running" ("scope mode") ScopeMode."Continuous" ("scope mode")] -> w399
              frame "Triggered" {
              }
              frame "Continuous" {
              }
            }
            n265 = Select(t=w399, s="Rumode", f=ScopeMode."Stopped" ("scope mode")) -> (s? t:f=w403:T18)
            n266 = Bundle By Name(cluster=w404, "scope mode"=w403) -> (w402:T17)
            n267 = case shown="\"Single\", \"Running\"" w403 {
              tunnel: w402 -> [w411 w418 w422]
              tunnel: [w412 w416 w423] -> w401
              frame "Single", "Running" {
                n268 = call "ToggleContinousMode.vi"("Cont Acquisition"=FALSE, "scope in"=w411) -> ("scope out"=w409:T17)  [unwired: 8 in, 1 out]
                n269 = call "ToggleAqcuisitionRunning_5782.vi"("Acquisition running"=TRUE, "scope in"=w409) -> ("scope out"=w413:T17)  [unwired: 8 in, 1 out]
                n270 = call "SendSWtrigger_5782.vi"("scope in"=w413) -> ("scope out"=w412:T17)  [unwired: 9 in, 1 out]
              }
              frame "Continuous" {
                n271 = call "ToggleAqcuisitionRunning_5782.vi"("Acquisition running"=TRUE, "scope in"=w418) -> ("scope out"=w417:T17)  [unwired: 8 in, 1 out]
                n272 = call "ToggleContinousMode.vi"("Cont Acquisition"=TRUE ("Acquisition running"), "scope in"=w417) -> ("scope out"=w416:T17)  [unwired: 8 in, 1 out]
              }
              frame "Stopped" {
                n273 = call "ToggleContinousMode.vi"("Cont Acquisition"=FALSE, "scope in"=w422) -> ("scope out"=w420:T17)  [unwired: 8 in, 1 out]
                n274 = call "ToggleAqcuisitionRunning_5782.vi"("Acquisition running"=FALSE, "scope in"=w420) -> ("scope out"=w423:T17)  [unwired: 8 in, 1 out]
              }
            }
          }
          event Value Change {
            n275 = event-data() -> ("CtlRef"=w427:refnum<vi>, "NewVal"=w425:bool)  [unwired: 1 in, 4 out]
            n276 = Search 1D Array(1D array=w428, element=w427) -> (index of element=w426:i32)  [unwired: 1 in]
            n277 = property on="Upper graph" class="WFGraph (strict)"("Active Plot"=w426, "Plot.Visible?"=w425) -> ()  [unwired: 2 in, 2 out]
            n278 = property on="Upper chart" class="WFChart (strict)"("Active Plot"=w426, "Plot.Visible?"=w425) -> ()  [unwired: 2 in, 2 out]
          }
          event Value Change {
            n279 = event-data() -> ("CtlRef"=w432:refnum<vi>, "NewVal"=w431:bool)  [unwired: 1 in, 4 out]
            n280 = local read "unwrap phase"() -> (w435:bool)
            n281 = Search 1D Array(1D array=w430, element=w432) -> (index of element=w439:i32)  [unwired: 1 in]
            n282 = Add(x=w439, y=2) -> (x+y=w437:i32)
            n283 = property on="freqdata" class="WFGraph (strict)"("Active Plot"=w439, "Plot.Visible?"=w431) -> ()  [unwired: 2 in, 2 out]
            n284 = Not(x=w435) -> (.not. x?=w434:bool)
            n285 = And(x=w435, y=w431) -> (x .and. y?=w436:bool)
            n286 = And(x=w434, y=w431) -> (x .and. y?=w433:bool)
            n287 = property on="Lower chart" class="WFChart (strict)"("Active Plot"=w439, "Plot.Visible?"=w433, "Active Plot"=w437, "Plot.Visible?"=w436) -> ()  [unwired: 2 in, 2 out]
          }
          event "unwrap phase": Value Change {
            n288 = event-data() -> ()  [unwired: 1 in, 6 out]
            n289 = local read "Ch1"() -> (w443:bool)
            n290 = local read "Ch0"() -> (w442:bool)
            n291 = Not(x="unwrap phase") -> (.not. x?=w448:bool)
            n292 = And(x=w443, y=w448) -> (x .and. y?=w447:bool)
            n293 = And(x=w442, y=w448) -> (x .and. y?=w446:bool)
            n294 = And(x=w442, y="unwrap phase") -> (x .and. y?=w445:bool)
            n295 = And(x=w443, y="unwrap phase") -> (x .and. y?=w444:bool)
            n296 = property on="Lower chart" class="WFChart (strict)"("Active Plot"=u32 0, "Plot.Visible?"=w447, "Active Plot"=u32 1, "Plot.Visible?"=w446) -> ()  [unwired: 2 in, 2 out]
            n297 = property on="Lower chart" class="WFChart (strict)"("Active Plot"=u32 2, "Plot.Visible?"=w445, "Active Plot"=u32 3, "Plot.Visible?"=w444) -> ()  [unwired: 2 in, 2 out]
          }
          event User Event {
            n298 = event-data() -> ("Sender"=w456:string, "Variant"=w455:variant, "driver status"=w454:T13)  [unwired: 1 in, 5 out]
            n299 = Unbundle By Name(w458) -> ("RemoteConnection"=w460:refnum<class "RemoteConnection.lvclass">)
            n300 = call "HandleRemoteMessage.vi"("driver status"=w454, "Message data"=w455, "Sender"=w456, "RemoteConnection in"=w460) -> ("RemoteConnection out"=w459:refnum<class "RemoteConnection.lvclass">)  [unwired: 6 in, 1 out]
            n301 = Bundle By Name(cluster=w458, "RemoteConnection"=w459) -> (w457:T17)
          }
          event "stop": Value Change {
            n302 = event-data() -> ()  [unwired: 1 in, 6 out]
          }
          event Value Change {
            n303 = event-data() -> ()  [unwired: 1 in, 6 out]
            n304 = case shown="\"V\"" "Unit" {
              tunnel: ["V" "dBV" "V^2"] -> w465
              frame "V" {
              }
              frame "dBV" {
              }
              frame "V^2" {
              }
            }
            n305 = Concatenate Strings("Amplitude [", w465, "]") -> (w463:string)
            n306 = property on="freqdata" class="WFGraph (strict)"("YScale.NameLbl.Text"=w463) -> ()  [unwired: 2 in, 2 out]
          }
          event "#bins": Value Change {
            n307 = event-data() -> ()  [unwired: 1 in, 6 out]
            n308 = local read "Upper chart"() -> (w474:dbl[][])
            n309 = local read "Window"() -> (w475:T8)
            n310 = local read "Unit"() -> (w476:T7)
            n311 = call "calc FFT.vi"("#bins"="#bins", "dt"=1e-06, "Unit"=w476, "Window"=w475, "data"=w474) -> ("Power Spectrum / PSD"=w473:cluster{"f0":dbl, "df":dbl, "magnitude":dbl[]}[])  [unwired: 6 in]
            n312 = local write "freqdata"(w473) -> ()
          }
          event "Zoom time X", "Zoom time Y": Value Change {
            n313 = event-data() -> ()  [unwired: 1 in, 6 out]
            n314 = control-ref of="Upper chart"() -> (w481:refnum<vi>)
            n315 = control-ref of="Upper graph"() -> (w482:refnum<vi>)
            n316 = call "setZoomTool.vi"("Zoom Y"="Zoom time Y", "Zoom  X"="Zoom time X", "reference"=w481) -> ()  [unwired: 9 in]
            n317 = call "setZoomTool.vi"("Zoom Y"="Zoom time Y", "Zoom  X"="Zoom time X", "reference"=w482) -> ()  [unwired: 9 in]
          }
          event "Zoom freq Y", "Zoom freq X": Value Change {
            n318 = event-data() -> ()  [unwired: 1 in, 6 out]
            n319 = control-ref of="Lower chart"() -> (w487:refnum<vi>)
            n320 = control-ref of="Lower graph"() -> (w486:refnum<vi>)
            n321 = control-ref of="freqdata"() -> (w488:refnum<vi>)
            n322 = call "setZoomTool.vi"("Zoom Y"="Zoom freq Y", "Zoom  X"="Zoom freq X", "reference"=w488) -> ()  [unwired: 9 in]
            n323 = call "setZoomTool.vi"("Zoom Y"="Zoom freq Y", "Zoom  X"="Zoom freq X", "reference"=w487) -> ()  [unwired: 9 in]
            n324 = call "setZoomTool.vi"("Zoom Y"="Zoom freq Y", "Zoom  X"="Zoom freq X", "reference"=w486) -> ()  [unwired: 9 in]
          }
          event Value Change {
            w492 = dbl[][] [] ("History Data")
            n325 = event-data() -> ()  [unwired: 1 in, 6 out]
            n326 = property on="Upper chart" class="WFChart (strict)"("History Data"=w492) -> ()  [unwired: 2 in, 2 out]
            n327 = property on="Lower chart" class="WFChart (strict)"("History Data"=w492) -> ()  [unwired: 2 in, 2 out]
            n328 = local write "freqdata"(cluster{"f0":dbl, "df":dbl, "magnitude":dbl[]}[] [] ("freqdata")) -> ()
            n329 = call "UpdateGraphs.vi"("Buffer mode"="Buffer", "Display mode"="Display", "Graph_refs"=w493) -> ()  [unwired: 9 in]
            n330 = property on="Zoom time X" class="Bool (strict)"("Val(Sgnl)"=TRUE ("Value (Signaling)")) -> ()  [unwired: 2 in, 2 out]
          }
        }
      }
      "stop 2" <- w118
    }
    frame Error {
    }
  }
  n331 = Unregister For Events(event registration refnum=w74) -> ()  [unwired: 1 in, 1 out]
  n332 = Unbundle By Name(w56) -> ("FPGA ref"=w82:T16, "RemoteConnection"=w17:refnum<class "RemoteConnection.lvclass">)
  n333 = flat-sequence {
    tunnel: w82 -> [w501]
    tunnel: w17 -> [w500]
    frame #0 {
      n334 = call "Close.vi"("RemoteConnection in"=w500) -> ()  [unwired: 9 in, 2 out]
      n335 = xnode "Close FPGA VI Reference"("FPGA VI Reference In"=w501) -> ()  [unwired: 1 in, 1 out]
      n336 = global write "global_stop.vi" "Stop"(TRUE ("Stop")) -> ()
    }
  }
